vi "Write VIs MAP.vi"(8 "error in (no error)":errorcluster, 10 "VIs MAP":map{T1, refnum<class "VI.lvclass">[]}(c390), 11 "Library in":refnum<class "Library.lvclass">) -> (0 "error out":errorcluster, 3 "Library out":refnum<class "Library.lvclass">)   [LabVIEW 2019, in "Panther Dashboard.lvlib" / "Library.lvclass"]
uses:
  Library.lvclass
  LabVIEWItem/Item Type--enum.ctl
  VI/VI.lvclass
  Library.lvclass/Library.ctl
  LabVIEWItem/LabVIEWItem.lvclass
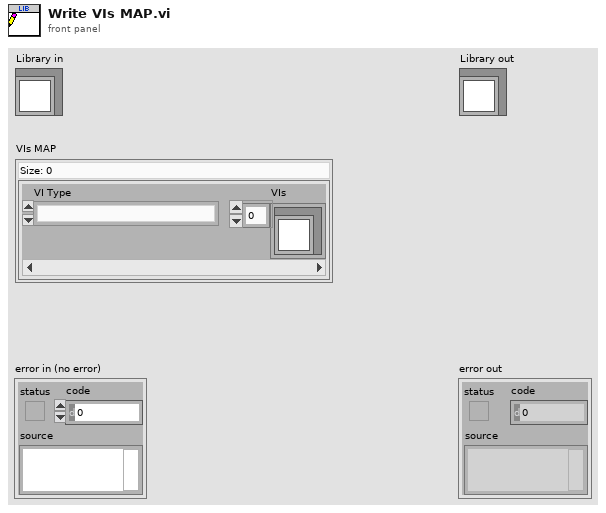
[diagram p1: front panel]
types:
  T1 = typedef "Panther Dashboard.lvlib/LabVIEWItem.lvclass/Item Type--enum.ctl" = enum16{"Requests", "Broadcasts", "Request and Wait for Reply", "Round Trip", "Public API VIs", "» Constant VIs", "» Error VIs", "Module", "Project"}
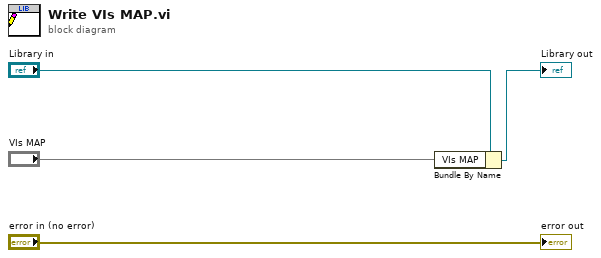
[diagram p0: block diagram]
diagram:
  n1 = Bundle By Name(cluster="Library in", "VIs MAP"="VIs MAP") -> (→"Library out":refnum<class "Library.lvclass">)
  "error out" <- "error in (no error)"
